vi "Pathfinder helper.vi"(9 "Types (string)":string[](array[string]), 10 "Data":string[](array[string])) -> ()   [LabVIEW 2020, in "Data.PG.lvclass"]
uses:
  Data.PG.lvclass
  <userlib>/_OpenG.lib/array/array.llb/Search 1D Array (String)__ogtk.vi
  <vilib>/ErrorRing/Error Ring.xnode
panel:
  in  "UNDO LAST VALUE":bool
  out "Paths":string[](array[string])
  out "String":string
  out "path_to_selected_column":string="llab_038:d001(TEST_TABLE--new_stuff(hippos))"
  out "table selected":string="TEST_TABLE"
  in  "columns_list":i32(listbox)=1
  in  "tables_list":i32(listbox)=34
  in  "STOP":bool
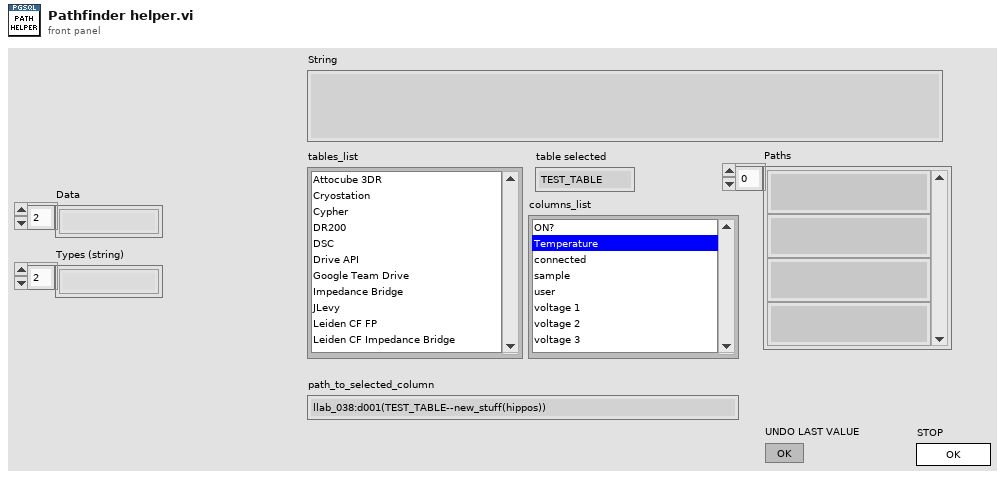
[diagram p1: front panel]
types:
  T1 = enum32{"Invalid", "Standard", "Closed", "Hidden", "Minimized", "Maximized"}
  T2 = enum32{"invalid app kind", "Development System", "Run Time System", "Student Edition", "Embedded LabVIEW", "Evaluation", "Custom"}
  T3 = cluster{"Core":cluster{"Current VI Reference":refnum<vi>, "Close Panel on Exit?":bool}, "Data.PG in":refnum<class "Data.PG.lvclass">, "connection info":cluster{"host":string, "port":string, "dbname":string, "user":string, "password":string}, "table names":string[], "table paths":string[], "column names":string[], "column units":string[], "column paths":string[], "new table name":string, "new column name":string, "new column data type":string, "new column units":string, "selected table":string, "selected column":string, "selected table path":string, "selected column path":string, "selected column units":string, "Paths array":string[], "Current Index":i32, "Data":string[], "Types (string)":string[]}
  T4 = cluster{"host":string, "port":string, "dbname":string, "user":string, "password":string}
  T5 = cluster{"Current VI Reference":refnum<vi>, "Close Panel on Exit?":bool}
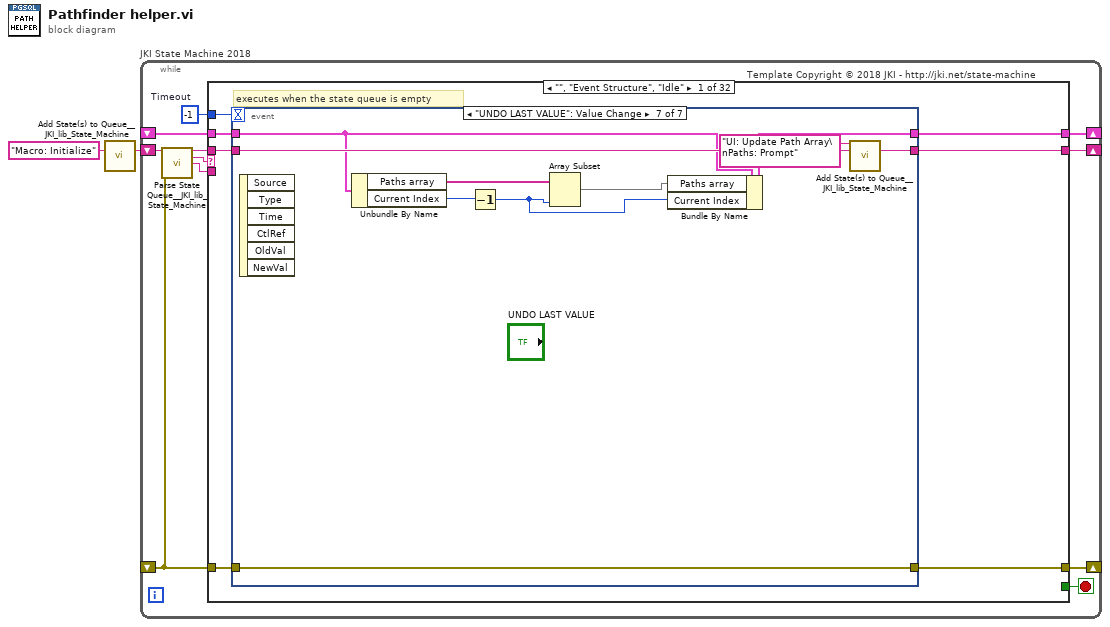
[diagram p0: block diagram]
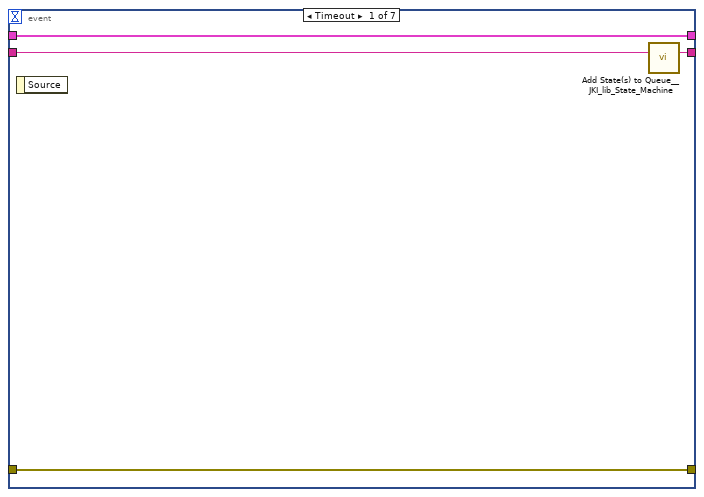
[diagram p2: hidden frame]
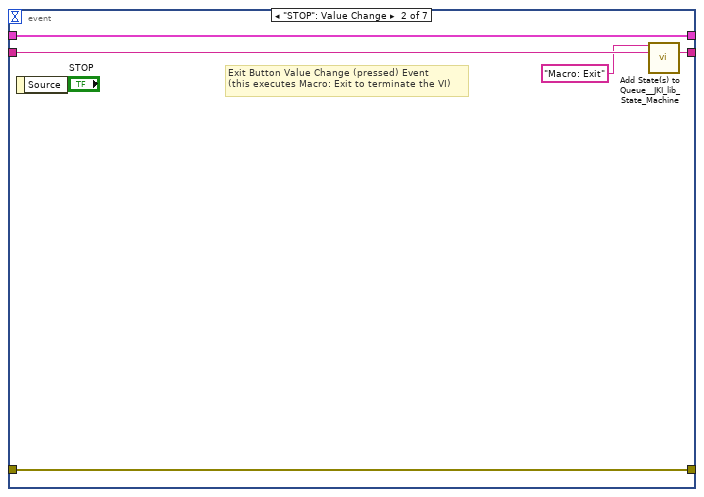
[diagram p3: hidden frame]
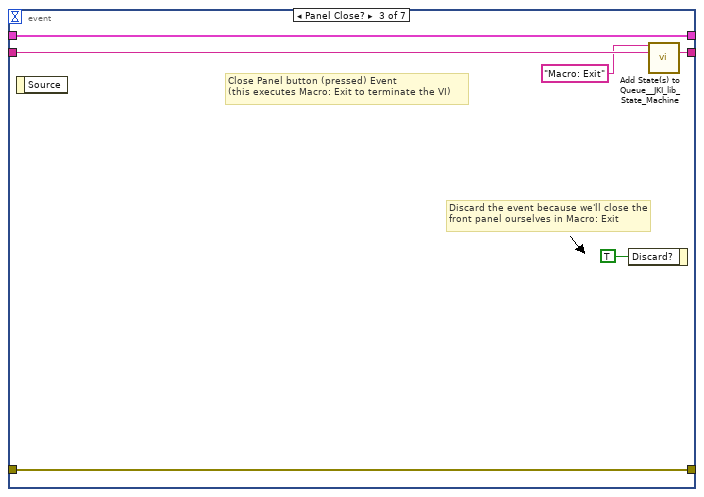
[diagram p4: hidden frame]
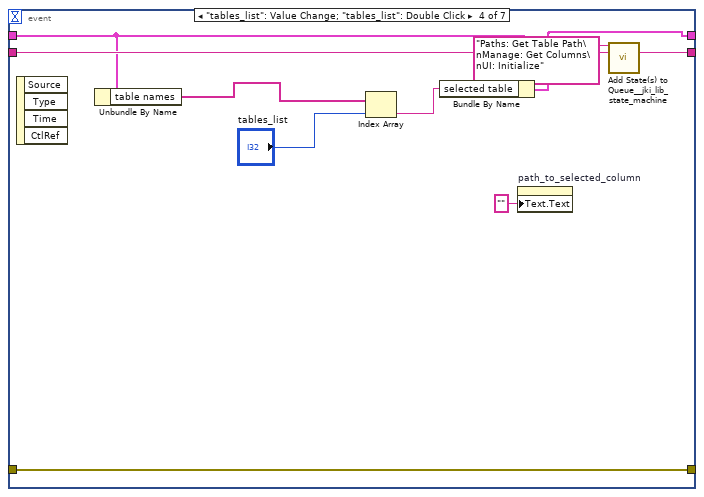
[diagram p5: hidden frame]
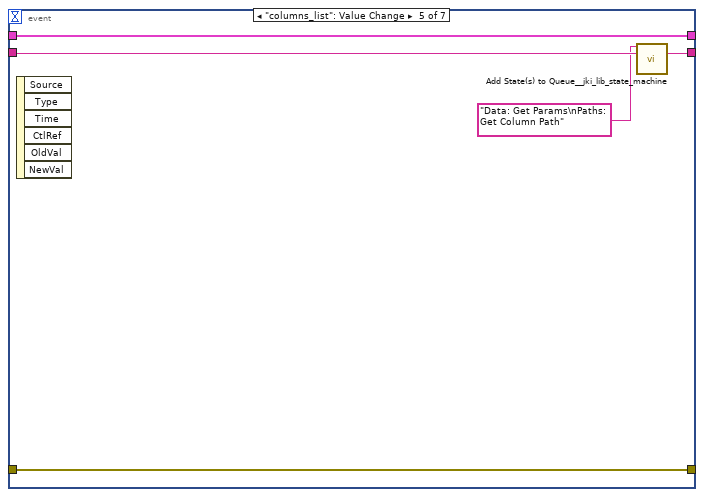
[diagram p6: hidden frame]
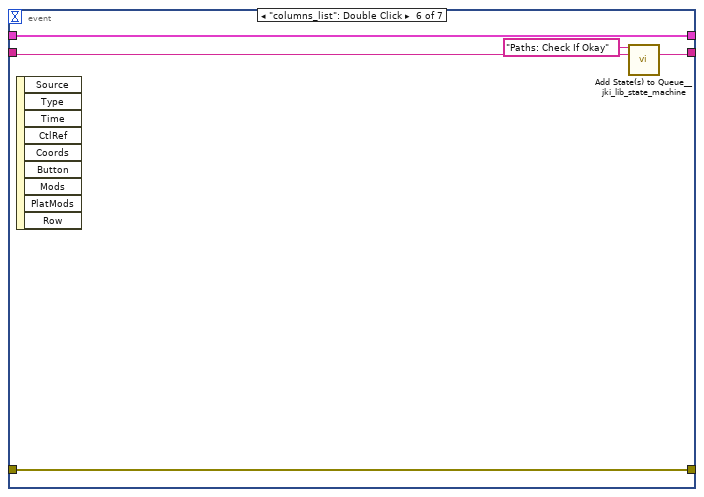
[diagram p7: hidden frame]
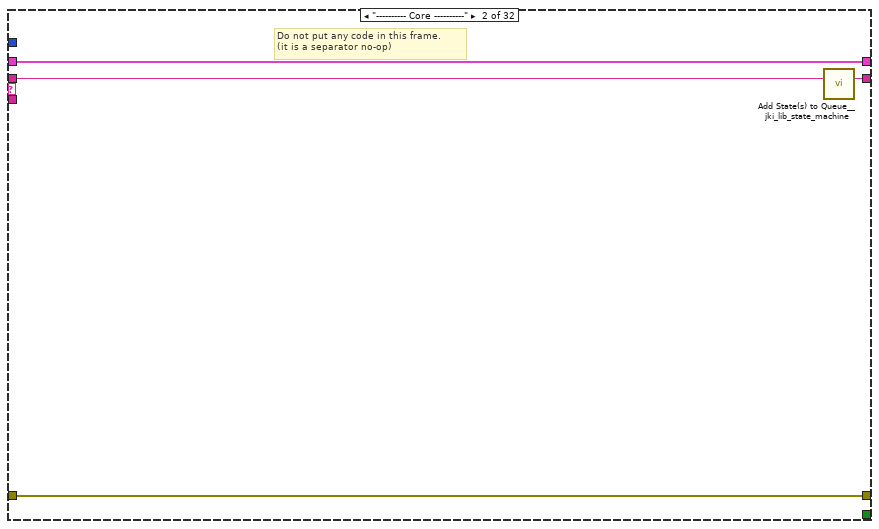
[diagram p8: hidden frame]
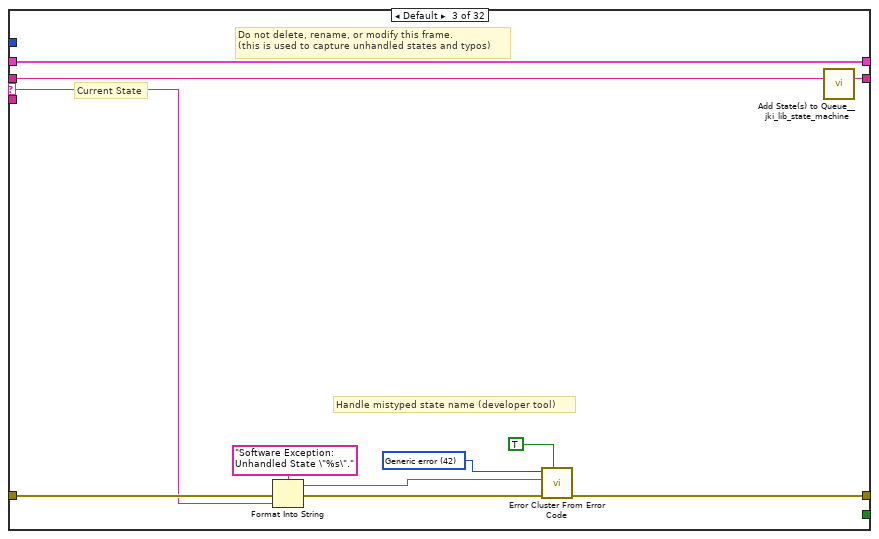
[diagram p9: hidden frame]
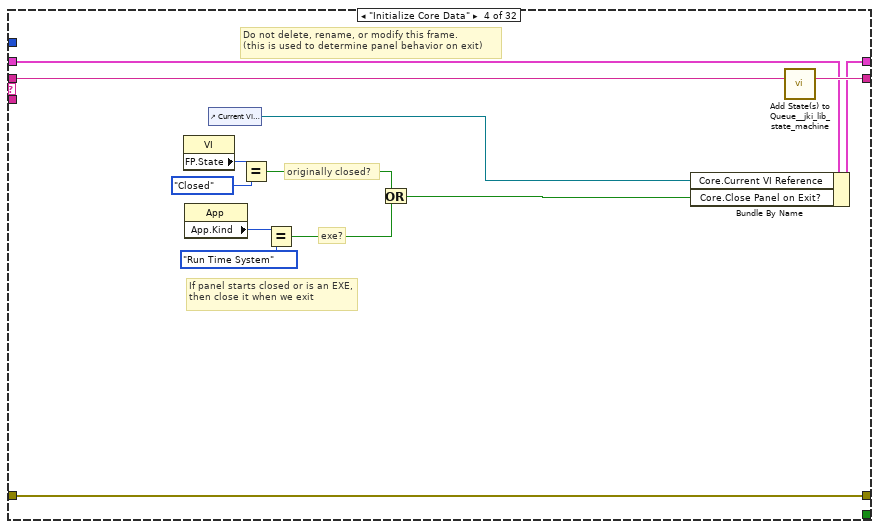
[diagram p10: hidden frame]
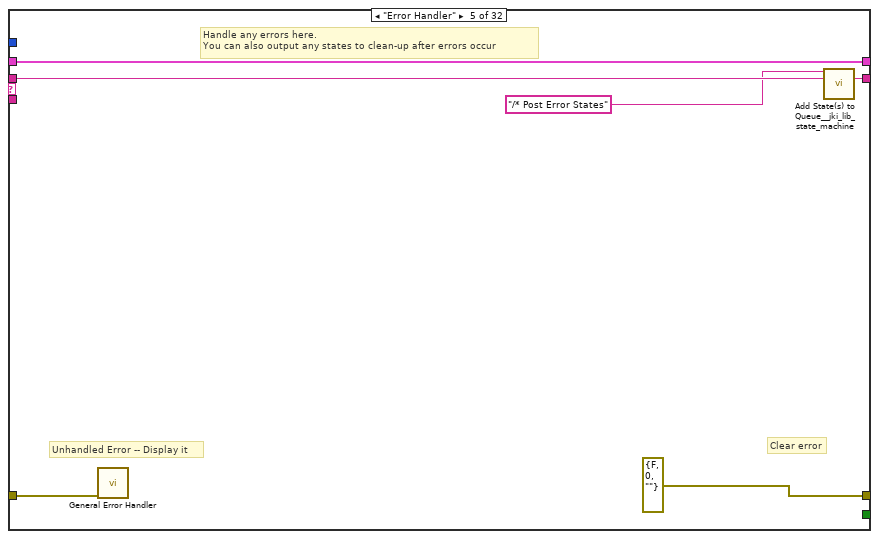
[diagram p11: hidden frame]
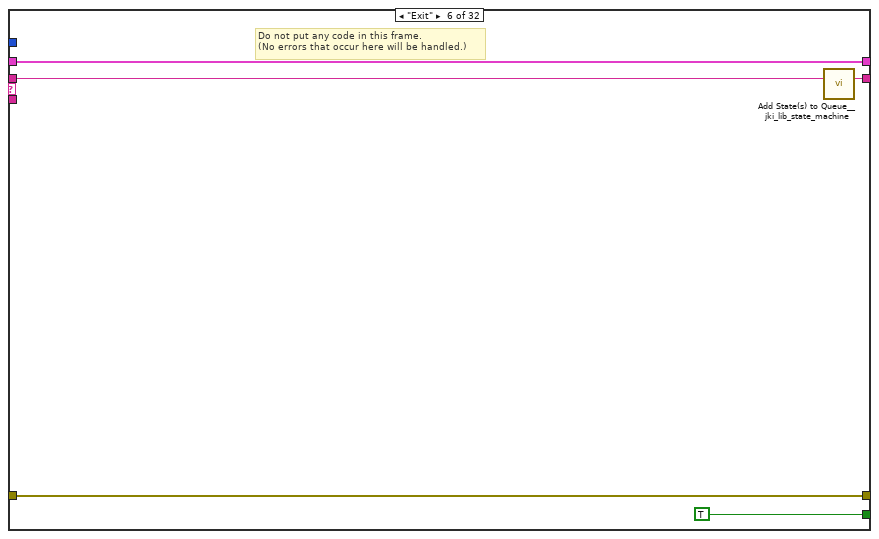
[diagram p12: hidden frame]
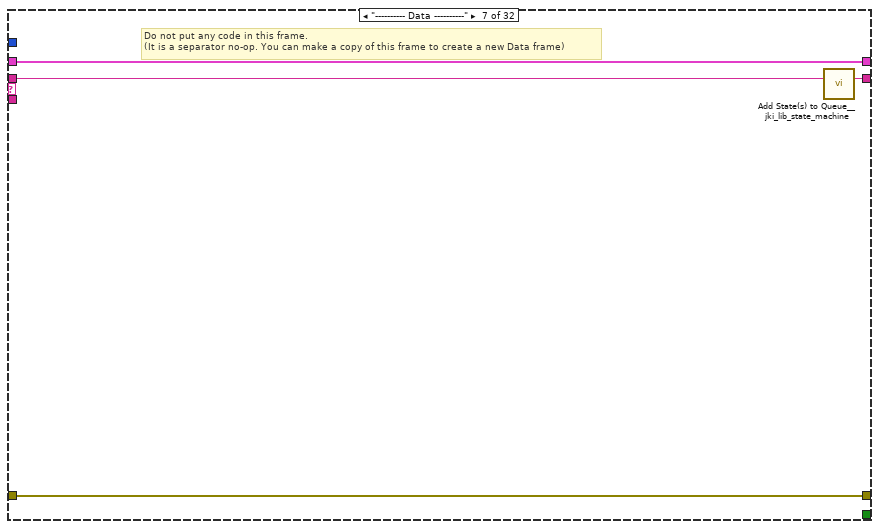
[diagram p13: hidden frame]
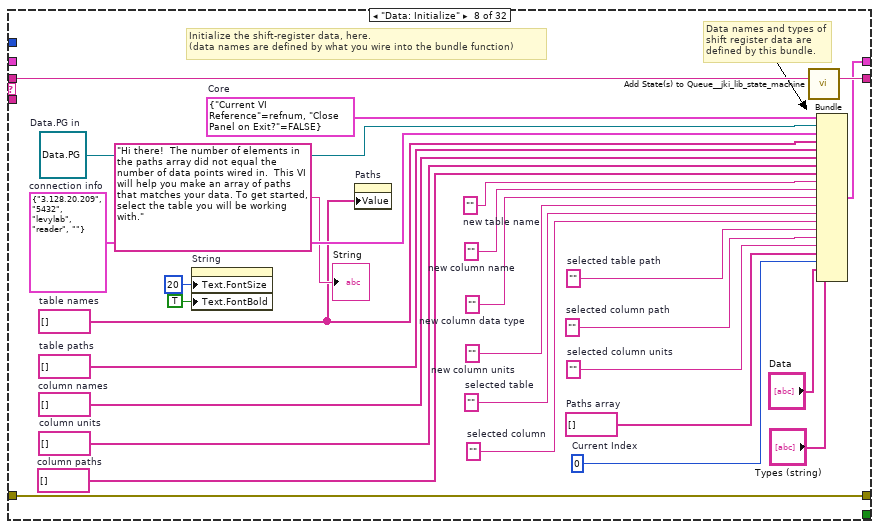
[diagram p14: hidden frame]
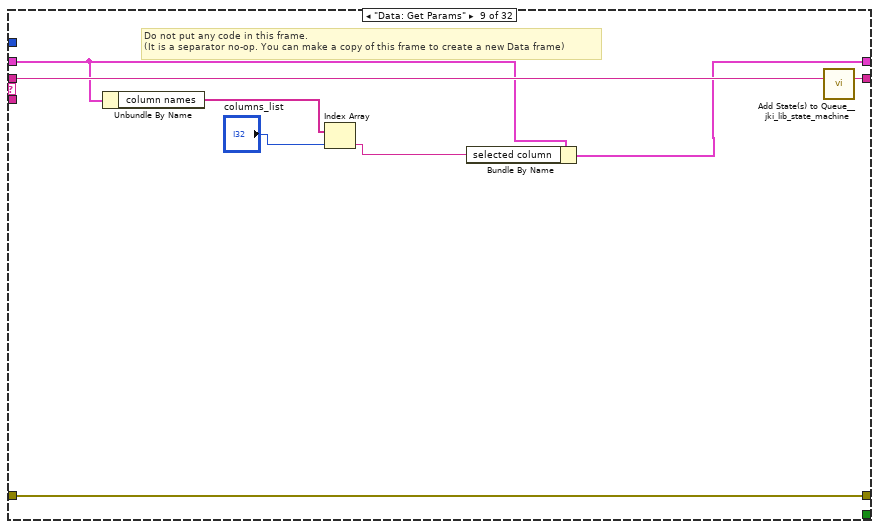
[diagram p15: hidden frame]
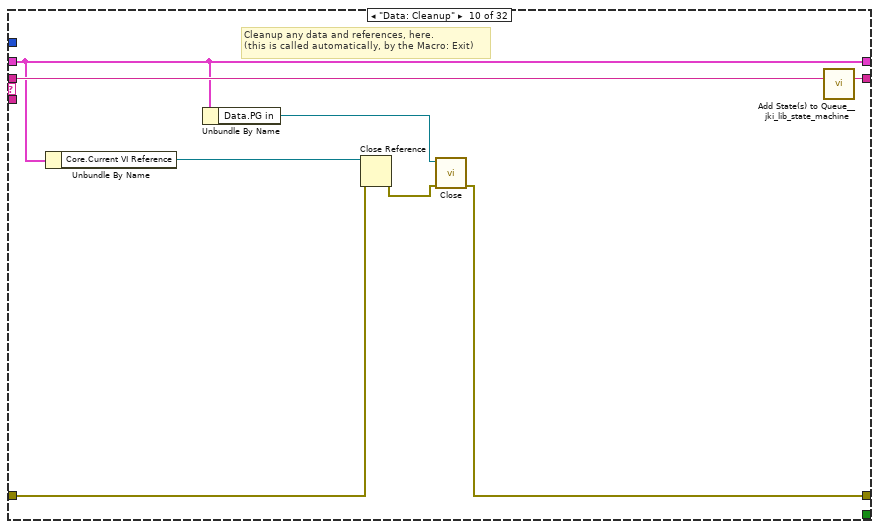
[diagram p16: hidden frame]
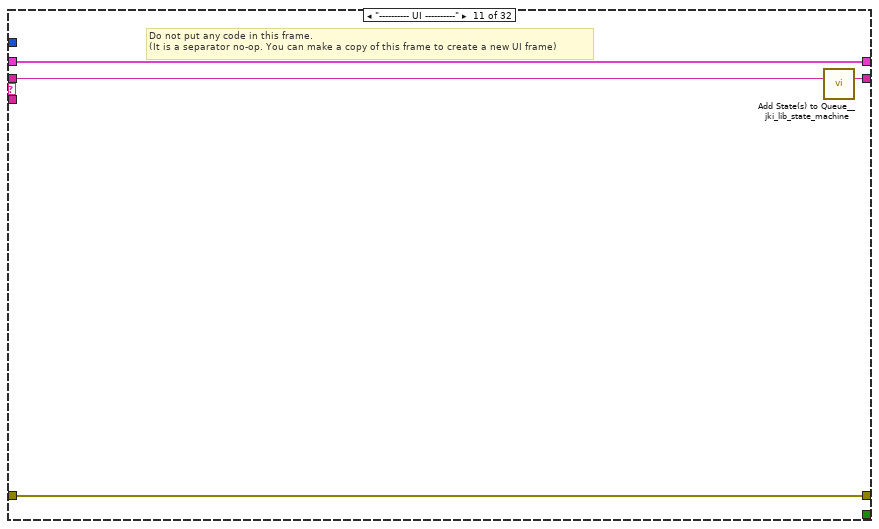
[diagram p17: hidden frame]
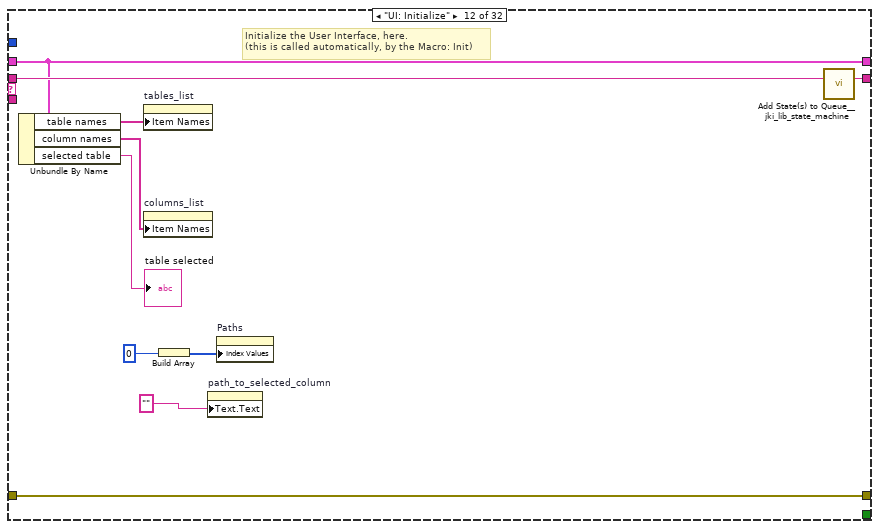
[diagram p18: hidden frame]
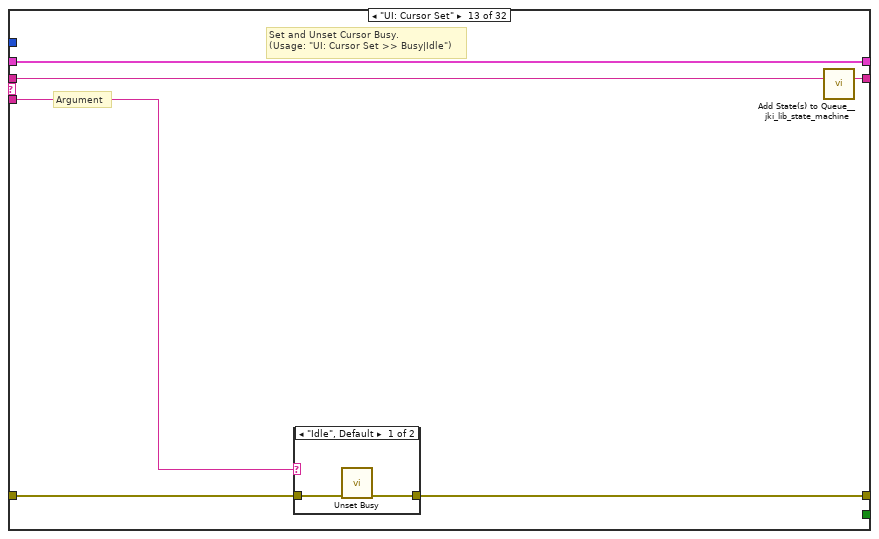
[diagram p19: hidden frame]
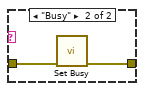
[diagram p20: hidden frame]
diagram:
  n1 = call <vilib>:"Add State(s) to Queue__JKI_lib_State_Machine.vi"("State(s) in (\"\")"="Macro: Initialize") -> ("States Out"=w2:string)  [unwired: 14 in]
  n2 = while "JKI State Machine 2018" {
    shift-right: [w6] -> _
    shift-left: _ -> [w5]
    shift-right: [w9] -> _
    shift-left: _ -> [w3]
    shift-right: [w8] -> _
    shift-left: w2 -> [w10]
    stop <- w7 stop-if-true
    w4 = -1  # Timeout
    # "Template Copyright © 2018 JKI - http://jki.net/state-machine"
    n3 = call <vilib>:"Parse State Queue__JKI_lib_State_Machine.vi"("State Queue"=w10, "Error In (no error)"=w3) -> ("Remaining States"=w12:string, "Current State"=w13:string, "Arguments"=w11:string)  [unwired: 11 in]
    n4 = case shown="\"\", \"Event Structure\", \"Idle\"" w13 {
      selector: w13 -> [_ _ w70 _ _ _ _ _ _ _ _ _ _ _ _ _ _ _ _ _ _ _ _ _ _ _ _ _ _ _ _ _]
      tunnel: w12 -> [w20 w69 w74 w93 w99 w104 w108 w136 w144 w152 w156 w166 w172 w183 w253 w258 w267 w271 w276 w286 w290 w303 w322 w326 w332 w341 w345 w358 w383 w394 w413 w448]
      tunnel: w11 -> [_ _ _ _ _ _ _ _ _ _ _ _ w167 w177 _ _ _ _ _ _ _ _ _ _ _ _ _ _ _ _ _ _]
      tunnel: w5 -> [w18 w66 w72 w86 w96 w102 w105 _ w140 w146 w153 w161 w170 w179 w250 w255 w264 w268 w273 w283 w287 w295 w311 w323 w330 w335 w342 w350 w376 w391 w407 w446]
      tunnel: [w17 w67 w76 w90 errorcluster {"status"=FALSE, "code"=0, "source"=""} ("error out") w101 w106 w133 w142 w147 w154 w164 w168 w180 w251 w256 w265 w269 w274 w284 w288 w297 w305 w324 w327 w336 w343 w346 w373 w392 w411 w423] -> w9
      tunnel: w3 -> [w16 w67 w75 w90 w95 w101 w106 w133 w142 w149 w154 w164 w169 w181 w251 w256 w265 w269 w274 w284 w288 w298 w306 w324 w328 w337 w343 w347 w374 w392 w411 w433]
      tunnel: [w19 w68 w73 w92 w98 w103 w107 w135 w143 w151 w155 w165 w171 w182 w252 w257 w266 w270 w275 w285 w289 w302 w321 w325 w331 w340 w344 w357 w382 w393 w412 w447] -> w8
      tunnel: [_ _ _ _ _ TRUE _ _ _ _ _ _ _ _ _ _ _ _ _ _ _ _ _ _ _ _ _ _ _ _ _ _] -> w7
      tunnel: [w15 w66 w72 w91 w96 w102 w105 w134 w141 w146 w153 w161 w170 w179 w250 w255 w264 w268 w273 w283 w287 w294 w310 w323 w330 w334 w342 w349 w375 w391 w406 w446] -> w6
      tunnel: w4 -> [w14 _ _ _ _ _ _ _ _ _ _ _ _ _ _ _ _ _ _ _ _ _ _ _ _ _ _ _ _ _ _ _]
      frame "", "Event Structure", "Idle" {
        # "executes when the state queue is empty"
        n5 = event shown="[6] \"UNDO LAST VALUE\": Value Change" {
          selector: _ -> [_ _ _ _ _ _ _]
          dyn-events: _ -> [_ _ _ _ _ _ _]
          timeout: w14 -> [_ _ _ _ _ _ _]
          tunnel: w20 -> [w24 w29 w35 w43 w48 w53 w63]
          tunnel: [w23 w28 w34 w44 w49 w54 w64] -> w19
          tunnel: w18 -> [w21 w26 w32 w39 w50 w52 w60]
          tunnel: [w22 w27 w33 w45 w46 w55 w65] -> w17
          tunnel: w16 -> [w22 w27 w33 w45 w46 w55 w65]
          tunnel: [w21 w26 w32 w38 w50 w52 w59] -> w15
          event Timeout {
            n6 = event-data() -> ()  [unwired: 1 in, 1 out]
            n7 = call <vilib>:"Add State(s) to Queue__JKI_lib_State_Machine.vi"("State(s) in (\"\")"=w24) -> ("States Out"=w23:string)  [unwired: 14 in]
          }
          event "STOP": Value Change {
            # "Exit Button Value Change (pressed) Event\n(this executes Macro: Exit to terminate the VI)"
            n8 = event-data() -> ()  [unwired: 1 in, 1 out]
            n9 = call <vilib>:"Add State(s) to Queue__JKI_lib_State_Machine.vi"("State(s) in Front (\"\")"="Macro: Exit", "State(s) in (\"\")"=w29) -> ("States Out"=w28:string)  [unwired: 13 in]
          }
          event Panel Close? {
            # "Discard the event because we'll close the front panel ourselves in Macro: Exit"
            # "Close Panel button (pressed) Event\n(this executes Macro: Exit to terminate the VI)"
            n10 = event-data() -> ()  [unwired: 1 in, 1 out]
            n11 = event-data("Discard?"=TRUE) -> ()  [unwired: 1 in, 1 out]
            n12 = call <vilib>:"Add State(s) to Queue__JKI_lib_State_Machine.vi"("State(s) in Front (\"\")"="Macro: Exit", "State(s) in (\"\")"=w35) -> ("States Out"=w34:string)  [unwired: 13 in]
          }
          event "tables_list": Value Change; "tables_list": Double Click {
            n13 = event-data() -> ()  [unwired: 1 in, 4 out]
            n14 = Unbundle By Name(w39) -> ("table names"=w40:string[])
            n15 = Index Array(array=w40, index="tables_list") -> (element=w37:string)
            n16 = Bundle By Name(cluster=w39, "selected table"=w37) -> (w38:T3)
            n17 = property on="path_to_selected_column" class="Str"("Text.Text"="") -> ()  [unwired: 2 in, 2 out]
            n18 = call <vilib>:"Add State(s) to Queue__jki_lib_state_machine.vi"("State(s) in Front (\"\")"="Paths: Get Table Path\nManage: Get Columns\nUI: Initialize" ("State(s) in Front (\"\")"), "State(s) in (\"\")"=w43) -> ("States Out"=w44:string)  [unwired: 13 in]
          }
          event "columns_list": Value Change {
            n19 = event-data() -> ()  [unwired: 1 in, 6 out]
            n20 = call <vilib>:"Add State(s) to Queue__jki_lib_state_machine.vi"("State(s) in Front (\"\")"="Data: Get Params\nPaths: Get Column Path", "State(s) in (\"\")"=w48) -> ("States Out"=w49:string)  [unwired: 13 in]
          }
          event "columns_list": Double Click {
            n21 = event-data() -> ()  [unwired: 1 in, 9 out]
            n22 = call <vilib>:"Add State(s) to Queue__jki_lib_state_machine.vi"("State(s) in Front (\"\")"="Paths: Check If Okay" ("State(s) in Front (\"\")"), "State(s) in (\"\")"=w53) -> ("States Out"=w54:string)  [unwired: 13 in]
          }
          event "UNDO LAST VALUE": Value Change {
            n23 = event-data() -> ()  [unwired: 1 in, 6 out]
            n24 = Unbundle By Name(w60) -> ("Paths array"=w61:string[], "Current Index"=w62:i32)
            n25 = Decrement(x=w62) -> (x-1=w58:i32)
            n26 = Array Subset(array=w61, length=w58) -> (w57:string[])  [unwired: 1 in]
            n27 = Bundle By Name(cluster=w60, "Paths array"=w57, "Current Index"=w58) -> (w59:T3)
            n28 = call <vilib>:"Add State(s) to Queue__JKI_lib_State_Machine.vi"("State(s) in Front (\"\")"="UI: Update Path Array\nPaths: Prompt" ("State(s) in Front (\"\")"), "State(s) in (\"\")"=w63) -> ("States Out"=w64:string)  [unwired: 13 in]
          }
        }
      }
      frame "---------- Core ----------" {
        # "Do not put any code in this frame.\n(it is a separator no-op)"
        n29 = call <vilib>:"Add State(s) to Queue__jki_lib_state_machine.vi"("State(s) in (\"\")"=w69) -> ("States Out"=w68:string)  [unwired: 14 in]
      }
      frame Default {
        w79 = 42 items=["No error", "Argument error", "Memory is full", "Out of zone", "End of file", "File already open", "Generic file I/O error", "File not found", "File permission error", "Disk is full", "Duplicate path", "Too many files open", "System feature not enabled", "Resource file not found", "Cannot add resource", "Resource not found", "Image not found", "Image memory error", "Pen does not exist", "Config type invalid", "Config token not found", "Config parse error", "Config memory error", "Bad external code format", "Bad external code offset", "External code not present", "Null window", "Destroy window error", "Null menu", "Print aborted", "Bad print record", "Print driver error", "Windows error during printing", "Memory error during printing", "Print dialog error", "Generic print error", "Invalid device refnum", "Device not found", "Device parameter error", "Device unit error", "Cannot open device", "Device call aborted", "Generic error", "Cancelled by user", "Object ID too low", "Object ID too high", "Object not in heap", "Unknown heap", "Unknown object (invalid DefProc)", "Unknown object (DefProc not in table)", "Message out of range", "Invalid (null) method", "Unknown message", "Manager call not supported", "Bad address", "Network operation in progress", "Network operation timed out", "Connection is busy", "Network attribute not supported", "Network error", "Address in use", "System out of memory", "Connection aborted", "Connection refused", "Not connected", "Already connected", "Connection closed", "Initialization error (interapplication manager)", "Bad occurrence", "Wait on unbound occurrence handler", "Occurrence queue overflow", "Datalog type conflict", "Unused", "Unrecognized type (interapplication manager)", "Memory corrupt", "Failed to make temporary DLL", "Old CIN version", "Drag socket not found", "Failed to load drop-object", "Failed to register OLE object", "Failed to release OLE object", "Format specifier type mismatch", "Unknown format specifier", "Too few format specifiers", "Too many format specifiers", "Scan failed", "Newer CIN version", "Error converting to variant", "Runtime menu error", "Password tampered", "Variant attribute not found", "Incompatible variant data type", "Event data is not available", "Event Store is not present", "Occurrence is not found", "Event Queue is not created", "Event info is not available", "Refnum passed is NULL", "Error retrieving Class GUID", "Error retrieving CoClass GUID", "Error retrieving TypeLib GUID.", "Bad built application magic bytes.", "Specific driver is different from the specific driver associated with the Logical Name.", "There is no session opened to the class driver.", "Max Error", "MAX - Error with config objects", "MAX - Error loading configuration", "MAX - Group not supported"]
        # "Current State"
        # "Do not delete, rename, or modify this frame.\n(this is used to capture unhandled states and typos)"
        # "Handle mistyped state name (developer tool)"
        n30 = Format Into String(format string="Software Exception: Unhandled State \"%s\"." ("message"), error in=w75, w70) -> (resulting string=w78:string, error out=w77:errorcluster)  [unwired: 1 in]
        n31 = call <vilib>:"Error Cluster From Error Code.vi"("show call chain? (False)"=TRUE, "error in (no error)"=w77, "error message (\"\")"=w78, "error code (0)"=w79) -> ("error out"=w76:errorcluster)  [unwired: 5 in]
        n32 = call <vilib>:"Add State(s) to Queue__jki_lib_state_machine.vi"("State(s) in (\"\")"=w74) -> ("States Out"=w73:string)  [unwired: 14 in]
      }
      frame "Initialize Core Data" {
        # "Do not delete, rename, or modify this frame.\n(this is used to determine panel behavior on exit)"
        # "originally closed?"
        # "exe?"
        # "If panel starts closed or is an EXE, then close it when we exit"
        n33 = property class="VI"() -> ("FP.State"=w83:T1)  [unwired: 2 in, 2 out]
        n34 = property class="App"() -> ("App.Kind"=w89:T2)  [unwired: 2 in, 2 out]
        n35 = control-ref of="Current VI Reference"() -> (w84:refnum<vi>)
        n36 = Equal?(x=w83, y=T1."Closed" ("Front Panel Window:State")) -> (x = y?=w81:bool)
        n37 = Equal?(x=w89, y=T2."Run Time System" ("Application:Kind")) -> (x = y?=w87:bool)
        n38 = Or(x=w81, y=w87) -> (x .or. y?=w85:bool)
        n39 = Bundle By Name(cluster=w86, "Core.Current VI Reference"=w84, "Core.Close Panel on Exit?"=w85) -> (w91:T3)
        n40 = call <vilib>:"Add State(s) to Queue__jki_lib_state_machine.vi"("State(s) in (\"\")"=w93) -> ("States Out"=w92:string)  [unwired: 14 in]
      }
      frame "Error Handler" {
        # "Unhandled Error -- Display it"
        # "Handle any errors here.\nYou can also output any states to clean-up after errors occur"
        # "Clear error"
        n41 = call <vilib>:"General Error Handler.vi"("error in (no error)"=w95) -> ()  [unwired: 10 in, 5 out]
        n42 = call <vilib>:"Add State(s) to Queue__jki_lib_state_machine.vi"("State(s) in Front (\"\")"="/* Post Error States", "State(s) in (\"\")"=w99) -> ("States Out"=w98:string)  [unwired: 13 in]
      }
      frame "Exit" {
        # "Do not put any code in this frame.\n(No errors that occur here will be handled.)"
        n43 = call <vilib>:"Add State(s) to Queue__jki_lib_state_machine.vi"("State(s) in (\"\")"=w104) -> ("States Out"=w103:string)  [unwired: 14 in]
      }
      frame "---------- Data ----------" {
        # "Do not put any code in this frame.\n(It is a separator no-op. You can make a copy of this frame to create a new Data frame)"
        n44 = call <vilib>:"Add State(s) to Queue__jki_lib_state_machine.vi"("State(s) in (\"\")"=w108) -> ("States Out"=w107:string)  [unwired: 14 in]
      }
      frame "Data: Initialize" {
        w115 = 0  # Current Index
        w116 = string[] []  # Paths array
        w117 = ""  # selected column units
        w118 = ""  # selected column path
        w119 = ""  # selected table path
        w120 = ""  # selected column
        w121 = ""  # selected table
        w122 = ""  # new column units
        w123 = ""  # new column data type
        w124 = ""  # new column name
        w125 = ""  # new table name
        w126 = string[] []  # column paths
        w127 = string[] []  # column units
        w128 = string[] []  # column names
        w129 = string[] []  # table paths
        w109 = string[] []  # table names
        w130 = T4 {"host"="3.128.20.209", "port"="5432", "dbname"="levylab", "user"="reader", "password"=""}  # connection info
        w131 = refnum<class "Data.PG.lvclass"> refnum  # Data.PG in
        w132 = T5 {"Current VI Reference"=refnum, "Close Panel on Exit?"=FALSE}  # Core
        # "Data names and types of shift register data are defined by this bundle."
        # "Initialize the shift-register data, here.\n(data names are defined by what you wire into the bundle function)"
        n45 = property on="String" class="Str"("Text.FontSize"=u32 20 ("Text.Font:Size"), "Text.FontBold"=TRUE ("Text.Font:Bold")) -> ()  [unwired: 2 in, 2 out]
        n46 = property on="Paths" class="Arr (strict)"("Value"=w109) -> ()  [unwired: 2 in, 2 out]
        n47 = call <vilib>:"Add State(s) to Queue__jki_lib_state_machine.vi"("State(s) in (\"\")"=w136) -> ("States Out"=w135:string)  [unwired: 14 in]
        n48 = Bundle("Core"=w132, "Data.PG in"=w131, "connection info"=w130, "table names"=w109, "table paths"=w129, "column names"=w128, "column units"=w127, "column paths"=w126, "new table name"=w125, "new column name"=w124, "new column data type"=w123, "new column units"=w122, "selected table"=w121, "selected column"=w120, "selected table path"=w119, "selected column path"=w118, "selected column units"=w117, "Paths array"=w116, "Current Index"=w115, "Data"="Data", "Types (string)"="Types (string)") -> (w134:T3)  [unwired: 1 in]
        "String" <- "Hi there!  The number of elements in the paths array did not equal the number of data points wired in.  This VI will help you make an array of paths that matches your data. To get started, select the table you will be working with." ("String")
      }
      frame "Data: Get Params" {
        # "Do not put any code in this frame.\n(It is a separator no-op. You can make a copy of this frame to create a new Data frame)"
        n49 = Unbundle By Name(w140) -> ("column names"=w138:string[])
        n50 = Index Array(array=w138, index="columns_list") -> (element=w137:string)
        n51 = Bundle By Name(cluster=w140, "selected column"=w137) -> (w141:T3)
        n52 = call <vilib>:"Add State(s) to Queue__jki_lib_state_machine.vi"("State(s) in (\"\")"=w144) -> ("States Out"=w143:string)  [unwired: 14 in]
      }
      frame "Data: Cleanup" {
        # "Cleanup any data and references, here.\n(this is called automatically, by the Macro: Exit)"
        n53 = Unbundle By Name(w146) -> ("Core.Current VI Reference"=w150:refnum<vi>)
        n54 = Unbundle By Name(w146) -> ("Data.PG in"=w145:refnum<class "Data.PG.lvclass">)
        n55 = Close Reference(reference=w150, error in (no error)=w149) -> (error out=w148:errorcluster)
        n56 = call-dynamic "Close.vi"("error in (no error)"=w148, "Data.PG in"=w145) -> ("error out"=w147:errorcluster)  [unwired: 8 in, 1 out]
        n57 = call <vilib>:"Add State(s) to Queue__jki_lib_state_machine.vi"("State(s) in (\"\")"=w152) -> ("States Out"=w151:string)  [unwired: 14 in]
      }
      frame "---------- UI ----------" {
        # "Do not put any code in this frame.\n(It is a separator no-op. You can make a copy of this frame to create a new UI frame)"
        n58 = call <vilib>:"Add State(s) to Queue__jki_lib_state_machine.vi"("State(s) in (\"\")"=w156) -> ("States Out"=w155:string)  [unwired: 14 in]
      }
      frame "UI: Initialize" {
        # "Initialize the User Interface, here.\n(this is called automatically, by the Macro: Init)"
        n59 = Unbundle By Name(w161) -> ("table names"=w163:string[], "column names"=w162:string[], "selected table"=→"table selected":string)
        n60 = property on="tables_list" class="LstBox (strict)"("Item Names"=w163) -> ()  [unwired: 2 in, 2 out]
        n61 = property on="columns_list" class="LstBox (strict)"("Item Names"=w162) -> ()  [unwired: 2 in, 2 out]
        n62 = Build Array(0) -> (w157:i32[])
        n63 = property on="path_to_selected_column" class="Str"("Text.Text"="") -> ()  [unwired: 2 in, 2 out]
        n64 = property on="Paths" class="Arr (strict)"("Index Values"=w157) -> ()  [unwired: 2 in, 2 out]
        n65 = call <vilib>:"Add State(s) to Queue__jki_lib_state_machine.vi"("State(s) in (\"\")"=w166) -> ("States Out"=w165:string)  [unwired: 14 in]
      }
      frame "UI: Cursor Set" {
        # "Argument"
        # "Set and Unset Cursor Busy.\n(Usage: \"UI: Cursor Set >> Busy|Idle\")"
        n66 = case shown="\"Idle\", Default" w167 {
          tunnel: w169 -> [w174 w176]
          tunnel: [w173 w175] -> w168
          frame "Idle", Default {
            n67 = call <vilib>:"Unset Busy.vi"("error in (no error)"=w174) -> ("error out"=w173:errorcluster)  [unwired: 10 in]
          }
          frame "Busy" {
            n68 = call <vilib>:"Set Busy.vi"("error in (no error)"=w176) -> ("error out"=w175:errorcluster)  [unwired: 9 in, 1 out]
          }
        }
        n69 = call <vilib>:"Add State(s) to Queue__jki_lib_state_machine.vi"("State(s) in (\"\")"=w172) -> ("States Out"=w171:string)  [unwired: 14 in]
      }
      frame "UI: Front Panel State" {
        # "Argument"
        # "Set Front Panel Open or Closed\n(Usage: \"UI: Front Panel State >> Open|Close\")"
        n70 = Unbundle By Name(w179) -> ("Core.Current VI Reference"=w178:refnum<vi>)
        n71 = case shown="\"Minimize\", \"Minimized\"" w177 {
          tunnel: w181 -> [w189 w204 w215 w228 w241]
          tunnel: [w191 w205 w217 w230 w243] -> w180
          tunnel: w178 -> [w190 w202 w216 w229 w242]
          frame "Open", "Standard", Default {
            w184 = T1."Standard" ("State")
            n72 = property class="VI"(reference=w190, error in=w189) -> (reference out=w187:refnum<vi>, error out=w188:errorcluster, "FP.State"=w186:T1)
            n73 = Not Equal?(x=w186, y=w184) -> (x != y?=w185:bool)
            n74 = case shown="True" w185 {
              tunnel: [w195 w197] -> w191
              tunnel: w188 -> [w194 w197]
              tunnel: w187 -> [w193 _]
              tunnel: w184 -> [w192 _]
              frame True {
                n75 = invoke class="VI" method="FP.Open"(reference=w193, error in=w194, "Activate"=TRUE, "State"=w192) -> (error out=w195:errorcluster)  [unwired: 1 in, 4 out]
              }
              frame False {
              }
            }
          }
          frame "Close", "Closed" {
            n76 = property class="VI"(reference=w202, error in=w204) -> (reference out=w201:refnum<vi>, error out=w203:errorcluster, "FP.State"=w199:T1)
            n77 = Not Equal?(x=w199, y=T1."Closed" ("Front Panel Window:State")) -> (x != y?=w198:bool)
            n78 = case shown="True" w198 {
              tunnel: [w206 w209] -> w205
              tunnel: w203 -> [w206 w208]
              tunnel: w201 -> [_ w207]
              frame False {
              }
              frame True {
                n79 = invoke class="VI" method="FP.Close"(reference=w207, error in=w208) -> (error out=w209:errorcluster)  [unwired: 1 in, 2 out]
              }
            }
          }
          frame "Hidden", "Hide" {
            w210 = T1."Hidden" ("State")
            n80 = property class="VI"(reference=w216, error in=w215) -> (reference out=w213:refnum<vi>, error out=w214:errorcluster, "FP.State"=w212:T1)
            n81 = Not Equal?(x=w212, y=w210) -> (x != y?=w211:bool)
            n82 = case shown="True" w211 {
              tunnel: [w221 w222] -> w217
              tunnel: w214 -> [w220 w222]
              tunnel: w213 -> [w219 _]
              tunnel: w210 -> [w218 _]
              frame True {
                n83 = invoke class="VI" method="FP.Open"(reference=w219, error in=w220, "State"=w218) -> (error out=w221:errorcluster)  [unwired: 2 in, 4 out]
              }
              frame False {
              }
            }
          }
          frame "Minimize", "Minimized" {
            w223 = T1."Minimized" ("State")
            n84 = property class="VI"(reference=w229, error in=w228) -> (reference out=w226:refnum<vi>, error out=w227:errorcluster, "FP.State"=w225:T1)
            n85 = Not Equal?(x=w225, y=w223) -> (x != y?=w224:bool)
            n86 = case shown="True" w224 {
              tunnel: [w234 w235] -> w230
              tunnel: w227 -> [w233 w235]
              tunnel: w226 -> [w232 _]
              tunnel: w223 -> [w231 _]
              frame True {
                n87 = invoke class="VI" method="FP.Open"(reference=w232, error in=w233, "State"=w231) -> (error out=w234:errorcluster)  [unwired: 2 in, 4 out]
              }
              frame False {
              }
            }
          }
          frame "Maximize", "Maximized" {
            w236 = T1."Maximized" ("State")
            n88 = property class="VI"(reference=w242, error in=w241) -> (reference out=w239:refnum<vi>, error out=w240:errorcluster, "FP.State"=w238:T1)
            n89 = Not Equal?(x=w238, y=w236) -> (x != y?=w237:bool)
            n90 = case shown="True" w237 {
              tunnel: [w247 w248] -> w243
              tunnel: w240 -> [w246 w248]
              tunnel: w239 -> [w245 _]
              tunnel: w236 -> [w244 _]
              frame True {
                n91 = invoke class="VI" method="FP.Open"(reference=w245, error in=w246, "State"=w244) -> (error out=w247:errorcluster)  [unwired: 2 in, 4 out]
              }
              frame False {
              }
            }
          }
        }
        n92 = call <vilib>:"Add State(s) to Queue__jki_lib_state_machine.vi"("State(s) in (\"\")"=w183) -> ("States Out"=w182:string)  [unwired: 14 in]
      }
      frame "UI: Update Path Array" {
        # "Do not put any code in this frame.\n(It is a separator no-op. You can make a copy of this frame to create a new UI frame)"
        n93 = Unbundle By Name(w250) -> ("Paths array"=→"Paths":string[])
        n94 = call <vilib>:"Add State(s) to Queue__jki_lib_state_machine.vi"("State(s) in (\"\")"=w253) -> ("States Out"=w252:string)  [unwired: 14 in]
      }
      frame "UI: Wait" {
        # "Do not put any code in this frame.\n(It is a separator no-op. You can make a copy of this frame to create a new UI frame)"
        n95 = Wait (ms)(milliseconds to wait=u32 15000) -> ()  [unwired: 1 out]
        n96 = call <vilib>:"Add State(s) to Queue__jki_lib_state_machine.vi"("State(s) in (\"\")"=w258) -> ("States Out"=w257:string)  [unwired: 14 in]
      }
      frame "UI: Finish" {
        # "Do not put any code in this frame.\n(It is a separator no-op. You can make a copy of this frame to create a new UI frame)"
        n97 = Unbundle By Name(w264) -> ("Paths array"=w263:string[])
        n98 = call <userlib>:"1D Array to String__ogtk.vi"("delimiter (Tab)"="\n", "Array of Strings"=w263) -> ("delimited string"=w262:string)  [unwired: 9 in]
        n99 = property on="String" class="Str"("Text.Text"="Great work! Your paths have been copied to your clipboard.  Find where you placed Insert.vi, wire a string constant to the control for paths, and paste the text from your clipboard into the string constant.  This VI will close after 15 seconds ") -> ()  [unwired: 2 in, 2 out]
        n100 = invoke class="App" method="Clipboard.Write"("Param 0"=w262) -> ()  [unwired: 3 in, 4 out]
        n101 = call <vilib>:"Add State(s) to Queue__jki_lib_state_machine.vi"("State(s) in Front (\"\")"="UI: Wait" ("State(s) in Front (\"\")"), "State(s) in (\"\")"=w267) -> ("States Out"=w266:string)  [unwired: 13 in]
      }
      frame "---------- Macro ----------" {
        # "Do not put any code in this frame.\n(It is a separator no-op. You can make a copy of this frame to create a new Macro frame)"
        n102 = call <vilib>:"Add State(s) to Queue__jki_lib_state_machine.vi"("State(s) in (\"\")"=w271) -> ("States Out"=w270:string)  [unwired: 14 in]
      }
      frame "Macro: Initialize" {
        w272 = "Data: Initialize\nInitialize Core Data\nConnection: Open\nManage: Get Tables\nUI: Initialize\nUI: Front Panel State >> Open"  # Data: Initialize Initialize Core Data Connection: Open Manage: Get Tables UI: Initialize UI: Front Panel State >> Open
        # "Initialization Macro\n(This is called once, when the VI starts)"
        n103 = call <vilib>:"Add State(s) to Queue__jki_lib_state_machine.vi"("State(s) in Front (\"\")"=w272, "State(s) in (\"\")"=w276) -> ("States Out"=w275:string)  [unwired: 13 in]
      }
      frame "Macro: Exit" {
        # "Exit Macro\n(This is called once, when the VI exits)"
        n104 = Unbundle By Name(w283) -> ("Core.Close Panel on Exit?"=w282:bool)
        n105 = Select(t="UI: Front Panel State >> Close", s=w282, f="") -> (s? t:f=w279:string)
        n106 = call <vilib>:"Add State(s) to Queue__jki_lib_state_machine.vi"("State(s) in (\"\")"=w279, "State(s) at Back (\"\")"="Data: Cleanup\nConnection: Close\nExit") -> ("States Out"=w277:string)  [unwired: 13 in]
        n107 = call <vilib>:"Add State(s) to Queue__jki_lib_state_machine.vi"("State(s) in Front (\"\")"=w277, "State(s) in (\"\")"=w286) -> ("States Out"=w285:string)  [unwired: 13 in]
      }
      frame "---------- Manage ----------" {
        # "Template Separator\n(You can make a copy of, or modify, this frame)"
        n108 = call <vilib>:"Add State(s) to Queue__jki_lib_state_machine.vi"("State(s) in (\"\")"=w290) -> ("States Out"=w289:string)  [unwired: 14 in]
      }
      frame "Manage: Get Tables" {
        # "Your code here.\n(You can make a copy of, or modify, this frame)"
        n109 = Unbundle By Name(w295) -> ("Data.PG in"=w301:refnum<class "Data.PG.lvclass">)
        n110 = call-dynamic "Test Read.vi"("error in (no error)"=w298, "command"="SELECT * FROM table_index ORDER BY name;", "Data.PG in"=w301) -> ("error out"=w297:errorcluster, "Result"=w299:string[][])  [unwired: 3 in, 4 out]
        n111 = Transpose 2D Array(2D array=w299) -> (transposed array=w296:string[][])
        n112 = Index Array(array=w296, index (row) #2=1 ("index (row)")) -> (element #1=w293:string[], element #2=w291:string[])  [unwired: 3 in]
        n113 = Bundle By Name(cluster=w295, "table names"=w293, "table paths"=w291) -> (w294:T3)
        n114 = call <vilib>:"Add State(s) to Queue__jki_lib_state_machine.vi"("State(s) in (\"\")"=w303) -> ("States Out"=w302:string)  [unwired: 14 in]
      }
      frame "Manage: Get Columns" {
        # "Your code here.\n(You can make a copy of, or modify, this frame)"
        n115 = Unbundle By Name(w311) -> ("Data.PG in"=w320:refnum<class "Data.PG.lvclass">, "selected table path"=w318:string)
        n116 = Format Into String(format string="SELECT * FROM %s_index WHERE name <>'time' ORDER BY name; ", w318) -> (resulting string=w317:string)  [unwired: 2 in, 1 out]
        n117 = call-dynamic "Test Read.vi"("error in (no error)"=w306, "command"=w317, "Data.PG in"=w320) -> ("error out"=w305:errorcluster, "Result"=w316:string[][])  [unwired: 3 in, 4 out]
        n118 = Transpose 2D Array(2D array=w316) -> (transposed array=w315:string[][])
        n119 = Index Array(array=w315, index (row) #1=0 ("index (row)"), index (row) #2=1 ("index (row)"), index (row) #3=2 ("index (row)")) -> (element #1=w309:string[], element #2=w308:string[], element #3=w307:string[])  [unwired: 3 in]
        n120 = Bundle By Name(cluster=w311, "column names"=w309, "column units"=w308, "column paths"=w307) -> (w310:T3)
        n121 = call <vilib>:"Add State(s) to Queue__jki_lib_state_machine.vi"("State(s) in Front (\"\")"="UI: Initialize\nPaths: Prompt" ("State(s) in Front (\"\")"), "State(s) in (\"\")"=w322) -> ("States Out"=w321:string)  [unwired: 13 in]
      }
      frame "---------- Connection ----------" {
        # "Template Separator\n(You can make a copy of, or modify, this frame)"
        n122 = call <vilib>:"Add State(s) to Queue__jki_lib_state_machine.vi"("State(s) in (\"\")"=w326) -> ("States Out"=w325:string)  [unwired: 14 in]
      }
      frame "Connection: Close" {
        # "Template Separator\n(You can make a copy of, or modify, this frame)"
        n123 = Unbundle By Name(w330) -> ("Data.PG in"=w329:refnum<class "Data.PG.lvclass">)
        n124 = call-dynamic "Close.vi"("error in (no error)"=w328, "Data.PG in"=w329) -> ("error out"=w327:errorcluster)  [unwired: 8 in, 1 out]
        n125 = call <vilib>:"Add State(s) to Queue__jki_lib_state_machine.vi"("State(s) in (\"\")"=w332) -> ("States Out"=w331:string)  [unwired: 14 in]
      }
      frame "Connection: Open" {
        # "Template Separator\n(You can make a copy of, or modify, this frame)"
        n126 = Unbundle By Name(w335) -> ("Data.PG in"=w339:refnum<class "Data.PG.lvclass">, "connection info"=w338:T4)
        n127 = call "Set Connection Info.vi"("error in (no error)"=w337, "connection info"=w338, "Data.PG in"=w339) -> ("error out"=w336:errorcluster, "Data.PG out"=w333:refnum<class "Data.PG.lvclass">)  [unwired: 7 in]
        n128 = Bundle By Name(cluster=w335, "Data.PG in"=w333) -> (w334:T3)
        n129 = call <vilib>:"Add State(s) to Queue__jki_lib_state_machine.vi"("State(s) in (\"\")"=w341) -> ("States Out"=w340:string)  [unwired: 14 in]
      }
      frame "---------- Paths ----------" {
        # "Template Separator\n(You can make a copy of, or modify, this frame)"
        n130 = call <vilib>:"Add State(s) to Queue__jki_lib_state_machine.vi"("State(s) in (\"\")"=w345) -> ("States Out"=w344:string)  [unwired: 14 in]
      }
      frame "Paths: Get Table Path" {
        # "Template Separator\n(You can make a copy of, or modify, this frame)"
        n131 = Unbundle By Name(w350) -> ("Data.PG in"=w355:refnum<class "Data.PG.lvclass">, "selected table"=w353:string)
        n132 = Format Into String(format string="SELECT path FROM table_index WHERE name='%s'", w353) -> (resulting string=w354:string)  [unwired: 2 in, 1 out]
        n133 = call-dynamic "Test Read.vi"("error in (no error)"=w347, "command"=w354, "Data.PG in"=w355) -> ("error out"=w346:errorcluster, "Result"=w352:string[][])  [unwired: 3 in, 4 out]
        n134 = Index Array(array=w352) -> (element=w351:string[])  [unwired: 2 in]
        n135 = Index Array(array=w351) -> (element=w348:string)  [unwired: 1 in]
        n136 = Bundle By Name(cluster=w350, "selected table path"=w348) -> (w349:T3)
        n137 = call <vilib>:"Add State(s) to Queue__jki_lib_state_machine.vi"("State(s) in (\"\")"=w358) -> ("States Out"=w357:string)  [unwired: 14 in]
      }
      frame "Paths: Get Column Path" {
        # "Template Separator\n(You can make a copy of, or modify, this frame)"
        n138 = Unbundle By Name(w376) -> ("Data.PG in"=w380:refnum<class "Data.PG.lvclass">, "selected table path"=w369:string, "selected column"=w372:string, "selected table"=w364:string, "selected column"=w362:string)
        n139 = Format Into String(format string="SELECT path,units FROM %s_index WHERE name='%s'", w369, w372) -> (resulting string=w379:string)  [unwired: 2 in, 1 out]
        n140 = call-dynamic "Test Read.vi"("error in (no error)"=w374, "command"=w379, "Data.PG in"=w380) -> ("error out"=w373:errorcluster, "Result"=w378:string[][])  [unwired: 3 in, 4 out]
        n141 = Index Array(array=w378) -> (element=w377:string[])  [unwired: 2 in]
        n142 = Index Array(array=w377, index #1=0 ("index"), index #2=1 ("index")) -> (element #1=w367:string, element #2=w360:string)
        n143 = Bundle By Name(cluster=w376, "selected column path"=w367, "selected column units"=w360) -> (w375:T3)
        n144 = Concatenate Strings(w369, ":" ("string"), w367, "(" ("string"), w364, "--" ("string"), w362, " (" ("string"), w360, "))" ("string")) -> (→"path_to_selected_column":string)
        n145 = call <vilib>:"Add State(s) to Queue__jki_lib_state_machine.vi"("State(s) in (\"\")"=w383) -> ("States Out"=w382:string)  [unwired: 14 in]
      }
      frame "Paths: Prompt" {
        # "Template Separator\n(You can make a copy of, or modify, this frame)"
        n146 = Unbundle By Name(w391) -> ("Current Index"=w386:i32, "Types (string)"=w388:string[], "Data"=w387:string[])
        n147 = Index Array(array=w388, index=w386) -> (element=w389:string)
        n148 = Index Array(array=w387, index=w386) -> (element=w385:string)
        n149 = Format Into String(format string="Element number --%d-- of data is of type --%s-- and has a value of --%s--.\nPlease double-click the column that stores this element", w386, w389, w385) -> (resulting string=w384:string)  [unwired: 2 in, 1 out]
        n150 = property on="String" class="Str"("Text.Text"=w384) -> ()  [unwired: 2 in, 2 out]
        n151 = call <vilib>:"Add State(s) to Queue__jki_lib_state_machine.vi"("State(s) in (\"\")"=w394) -> ("States Out"=w393:string)  [unwired: 14 in]
      }
      frame "Paths: Add Path" {
        # "Template Separator\n(You can make a copy of, or modify, this frame)"
        n152 = property on="path_to_selected_column" class="Str"() -> ("Text.Text"=w409:string)  [unwired: 2 in, 2 out]
        n153 = Unbundle By Name(w407) -> ("Paths array"=w410:string[], "Current Index"=w404:i32, "Data"=w405:string[])
        n154 = Increment(x=w404) -> (x+1=w395:i32)
        n155 = Array Size(array=w405) -> (size(s)=w403:i32)
        n156 = Equal?(x=w395, y=w403) -> (x = y?=w402:bool)
        n157 = case shown="False" w402 {
          tunnel: w395 -> [w419 w422]
          tunnel: [w419 w420] -> w398
          tunnel: ["UI: Update Path Array\nPaths: Prompt" ("State(s) in Front (\"\")") "UI: Update Path Array\nUI: Finish\nMacro: Exit" ("State(s) in Front (\"\")")] -> w401
          frame False {
          }
          frame True {
            n158 = Decrement(x=w422) -> (x-1=w420:i32)
          }
        }
        n159 = Insert Into Array(array=w410, new element=w409) -> (w408:string[])  [unwired: 1 in]
        n160 = Greater?(x=w395, y=4) -> (0:w400:bool)
        n161 = case shown="True" w400 {
          tunnel: w395 -> [_ w417]
          tunnel: [0 w415] -> w396
          frame False {
          }
          frame True {
            n162 = Subtract(x=w417, y=4) -> (x-y=w415:i32)
          }
        }
        n163 = Bundle By Name(cluster=w407, "Paths array"=w408, "Current Index"=w398) -> (w406:T3)
        n164 = Build Array(w396) -> (w397:i32[])
        n165 = property on="Paths" class="Arr (strict)"("Index Values"=w397) -> ()  [unwired: 2 in, 2 out]
        n166 = call <vilib>:"Add State(s) to Queue__jki_lib_state_machine.vi"("State(s) in Front (\"\")"=w401, "State(s) in (\"\")"=w413) -> ("States Out"=w412:string)  [unwired: 13 in]
      }
      frame "Paths: Check If Okay" {
        # "Template Separator\n(You can make a copy of, or modify, this frame)"
        n167 = Unbundle By Name(w446) -> ("Paths array"=w445:string[], "Types (string)"=w437:string[], "Current Index"=w436:i32)
        n168 = property on="path_to_selected_column" class="Str"() -> ("Text.Text"=w426:string)  [unwired: 2 in, 2 out]
        n169 = call-poly <userlib>:"Search Array__ogtk.vi"("Array"=w445, "Element Data"=w426) -> ("Indices of Elements"=w444:i32[])  [unwired: 7 in]
        n170 = Search/Split String(string=w426, search string/char (-)=":") -> (match + rest of string=w425:string)  [unwired: 1 in, 2 out]
        n171 = Index Array(array=w437, index=w436) -> (element=w435:string)
        n172 = Array Size(array=w444) -> (size(s)=w443:i32)
        n173 = String Subset(string=w425, offset (0)=1, length (rest)=1 ("length (rest)")) -> (substring=w438:string)
        n174 = Equal To 0?(x=w443) -> (x = 0?=w442:bool)
        n175 = case shown="\"v\"" w438 {
          tunnel: w435 -> [_ w456 w466 w476 w486]
          tunnel: [w449 w455 w465 w475 w485] -> w434
          frame "False", Default {
            n176 = xnode "Error Ring"() -> ("error out"=w449:errorcluster)
          }
          frame "v" {
            n177 = case shown="\"string\"" w456 {
              tunnel: [w457 w463] -> w455
              frame "False", Default {
                n178 = xnode "Error Ring"() -> ("error out"=w457:errorcluster)
              }
              frame "string" {
                n179 = xnode "Error Ring"() -> ("error out"=w463:errorcluster)
              }
            }
          }
          frame "b" {
            n180 = case shown="\"boolean\"" w466 {
              tunnel: [w467 w473] -> w465
              frame "False", Default {
                n181 = xnode "Error Ring"() -> ("error out"=w467:errorcluster)
              }
              frame "boolean" {
                n182 = xnode "Error Ring"() -> ("error out"=w473:errorcluster)
              }
            }
          }
          frame "d" {
            n183 = case shown="\"False\", Default" w476 {
              tunnel: [w477 w483] -> w475
              frame "False", Default {
                n184 = xnode "Error Ring"() -> ("error out"=w477:errorcluster)
              }
              frame "double", "integer" {
                n185 = xnode "Error Ring"() -> ("error out"=w483:errorcluster)
              }
            }
          }
          frame "i" {
            n186 = case shown="\"False\", Default" w486 {
              tunnel: [w487 w493] -> w485
              frame "False", Default {
                n187 = xnode "Error Ring"() -> ("error out"=w487:errorcluster)
              }
              frame "integer" {
                n188 = xnode "Error Ring"() -> ("error out"=w493:errorcluster)
              }
            }
          }
        }
        n189 = case shown="False" w442 {
          tunnel: [w495 w501] -> w432
          frame False {
            n190 = xnode "Error Ring"() -> ("error out"=w495:errorcluster)
          }
          frame True {
            n191 = xnode "Error Ring"() -> ("error out"=w501:errorcluster)
          }
        }
        n192 = Merge Errors(w432, w434, w433) -> (w431:errorcluster)
        n193 = call <vilib>:"Simple Error Handler.vi"("error in (no error)"=w431) -> ("error?"=w428:bool, "error out"=w424:errorcluster)  [unwired: 4 in, 3 out]
        n194 = Select(t="", s=w428, f="Paths: Add Path") -> (s? t:f=w427:string)
        n195 = call <vilib>:"Clear Errors.vi"("error in (no error)"=w424) -> ("error out"=w423:errorcluster)  [unwired: 5 in, 1 out]
        n196 = call <vilib>:"Add State(s) to Queue__jki_lib_state_machine.vi"("State(s) in Front (\"\")"=w427, "State(s) in (\"\")"=w448) -> ("States Out"=w447:string)  [unwired: 13 in]
      }
    }
  }
